vi "Neslab Command Build 03.vi"(6 "Set Value":dbl format="%.2f", 7 "Command":T1(ring), 8 "Addr LSB":u8=1 format="%02x", 9 "Addr MSB":u8 format="%02x") -> (0 "Chksum":u8 format="%02x", 2 "Cmd Arr":u8[](array[numeric]) format="%02x", 3 "Cmd Str":string)   [LabVIEW 2023]
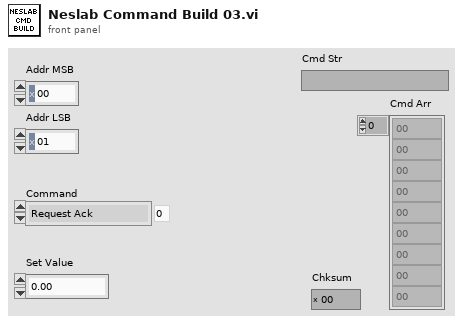
[diagram p1: front panel]
types:
  T1 = enum16{"Request Ack", "Set Setpoint", "Set Lo Limit", "Set Hi Limit", "Set Prop Band 0-99.9", "Set Integral 0-9.99", "Set Derivative 0-5.0", "Read Int Temp", "Read Ext Temp", "Read Setpoint", "Read Low Limit", "Read High Limit", "Read Prop Band", "Read Integral", "Read Derivative "}
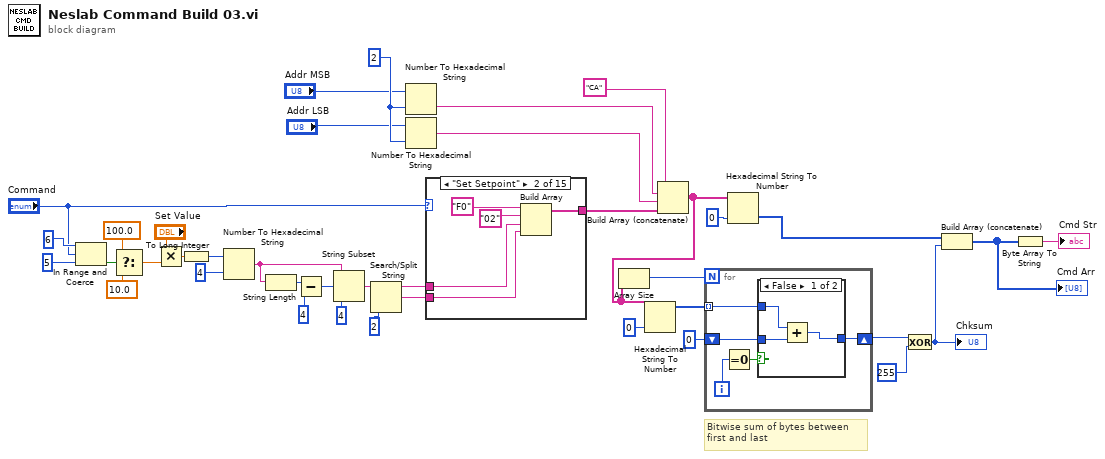
[diagram p0: block diagram]
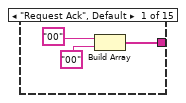
[diagram p3: hidden frame]
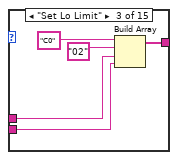
[diagram p4: hidden frame]
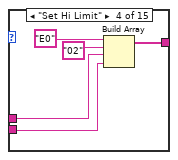
[diagram p5: hidden frame]
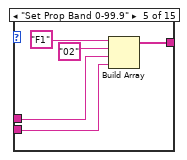
[diagram p6: hidden frame]
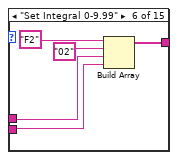
[diagram p7: hidden frame]
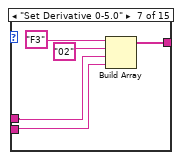
[diagram p8: hidden frame]
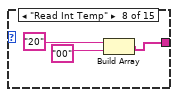
[diagram p9: hidden frame]
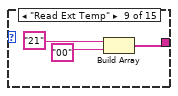
[diagram p10: hidden frame]
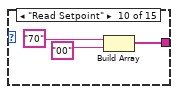
[diagram p11: hidden frame]
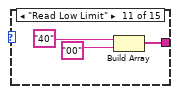
[diagram p12: hidden frame]
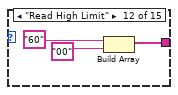
[diagram p13: hidden frame]
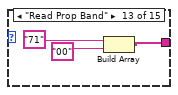
[diagram p14: hidden frame]
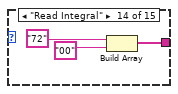
[diagram p15: hidden frame]
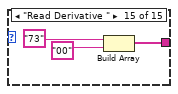
[diagram p16: hidden frame]
diagram:
  w5 = i16 2 ("width (-)")
  # "Bitwise sum of bytes between \nfirst and last"
  n1 = In Range and Coerce(upper limit=6 ("y"), x="Command", lower limit=5 ("y")) -> (In Range?=w7:bool)  [unwired: 1 out]
  n2 = Select(t=100.0 ("y"), s=w7, f=10.0) -> (s? t:f=w14:dbl)
  n3 = Multiply(x="Set Value", y=w14) -> (x*y=w29:dbl)
  n4 = To Long Integer(number=w29) -> (32bit integer=w13:i32)
  n5 = Number To Hexadecimal String(1:i16 4 ("width (-)"), 2:w13) -> (0:w32:string)
  n6 = String Length(string=w32) -> (length=w35:i32)
  n7 = Subtract(x=w35, y=4) -> (x-y=w34:i32)
  n8 = String Subset(string=w32, offset (0)=w34, length (rest)=4 ("length (rest)")) -> (substring=w30:string)
  n9 = Search/Split String(string=w30, offset (0)=2) -> (substring before match=w11:string, match + rest of string=w10:string)  [unwired: 1 in, 1 out]
  n10 = Number To Hexadecimal String(1:w5, 2:"Addr MSB") -> (0:w2:string)
  n11 = Number To Hexadecimal String(1:w5, 2:"Addr LSB") -> (0:w1:string)
  n12 = case shown="\"Set Setpoint\"" "Command" {
    tunnel: [w40 w45 w48 w53 w58 w63 w70 w73 w76 w79 w82 w85 w88 w91 w94] -> w27
    tunnel: w11 -> [_ w44 w50 w55 w60 w65 w69 _ _ _ _ _ _ _ _]
    tunnel: w10 -> [_ w43 w49 w54 w59 w64 w68 _ _ _ _ _ _ _ _]
    frame "Request Ack", Default {
      n13 = Build Array("00", "00") -> (w40:string[])
    }
    frame "Set Setpoint" {
      n14 = Build Array("F0", "02", w44, w43) -> (w45:string[])
    }
    frame "Set Lo Limit" {
      n15 = Build Array("C0", "02", w50, w49) -> (w48:string[])
    }
    frame "Set Hi Limit" {
      n16 = Build Array("E0", "02", w55, w54) -> (w53:string[])
    }
    frame "Set Prop Band 0-99.9" {
      n17 = Build Array("F1", "02", w60, w59) -> (w58:string[])
    }
    frame "Set Integral 0-9.99" {
      n18 = Build Array("F2", "02", w65, w64) -> (w63:string[])
    }
    frame "Set Derivative 0-5.0" {
      n19 = Build Array("F3", "02", w69, w68) -> (w70:string[])
    }
    frame "Read Int Temp" {
      n20 = Build Array("20", "00") -> (w73:string[])
    }
    frame "Read Ext Temp" {
      n21 = Build Array("21", "00") -> (w76:string[])
    }
    frame "Read Setpoint" {
      n22 = Build Array("70", "00") -> (w79:string[])
    }
    frame "Read Low Limit" {
      n23 = Build Array("40", "00") -> (w82:string[])
    }
    frame "Read High Limit" {
      n24 = Build Array("60", "00") -> (w85:string[])
    }
    frame "Read Prop Band" {
      n25 = Build Array("71", "00") -> (w88:string[])
    }
    frame "Read Integral" {
      n26 = Build Array("72", "00") -> (w91:string[])
    }
    frame "Read Derivative " {
      n27 = Build Array("73", "00") -> (w94:string[])
    }
  }
  n28 = Build Array (concatenate)("CA", w2, w1, w27) -> (w21:string[])
  n29 = Array Size(array=w21) -> (size(s)=w12:i32)
  n30 = Hexadecimal String To Number(string=w21, default (0uL)=u8 0 ("default (0 U32)")) -> (number=w26:u8[])  [unwired: 1 in, 1 out]
  n31 = for {
    N: w12 -> [_]
    tunnel: w26 -> [w99] mode=indexing
    shift-right: [w97] -> w22
    shift-left: u8 0 -> [w98]
    i -> [w101]
    n32 = Equal To 0?(x=w101) -> (x = 0?=w100:bool)
    n33 = case shown="False" w100 {
      tunnel: w99 -> [w103 _]
      tunnel: w98 -> [w104 w105]
      tunnel: [w102 w105] -> w97
      frame False {
        n34 = Add(x=w103, y=w104) -> (x+y=w102:u8)
      }
      frame True {
      }
    }
  }
  n35 = Hexadecimal String To Number(string=w21, default (0uL)=u8 0 ("default (0 U32)")) -> (number=w20:u8[])  [unwired: 1 in, 1 out]
  n36 = Exclusive Or(1:u8 255 ("y"), 2:w22) -> (0:w19:u8)
  "Chksum" <- w19
  n37 = Build Array (concatenate)(w20, w19) -> (w18:u8[])
  "Cmd Arr" <- w18
  n38 = Byte Array To String(unsigned byte array=w18) -> (string=→"Cmd Str":string)
